vi "PressureMultiplexer global.vi"() -> ()   [LabVIEW 2015]
panel:
  in  "Data rate (Hz)":dbl
  out "First run":bool=TRUE
  in  "VISA resource name":refnum<visa-resource-name>
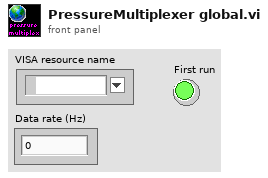
[diagram p1: front panel]
diagram:
